vi "Handle Error.vi"(8 "error in (no error)":errorcluster, 11 "IMAQdx Actor in":refnum<class "IMAQdx Actor.lvclass">) -> (0 "error out":errorcluster, 2 "stop actor?":bool=TRUE, 3 "IMAQdx Actor out":refnum<class "IMAQdx Actor.lvclass">)   [LabVIEW 2020, in "IMAQdx Actor.lvlib" / "IMAQdx Actor.lvclass"]
doc: "(<B>Filename</B>: Actor Framework.lvlib:Actor.lvclass:Handle Error.vi)\n\nDefines how the actor handles an error that occurred while processing a message. By default, this method does nothing except stop the actor."
uses:
  IMAQdx Actor.lvclass
  C:/Users/AlexK/work/LabVIEW Programme/POLARIS CAM Log Abw und E/Submodules/HIJ Vision/Camera Actors/Camera Actor/Camera Actor/Camera Actor.lvclass
  C:/Program Files (x86)/National Instruments/LabVIEW 2020/vi.lib/ActorFramework/Actor/Actor.lvclass
  Camera Actor/Camera Actor/Camera Actor.lvclass/Camera Actor.ctl
  Camera Actor/Camera Actor/Operation Mode.ctl
  Report Error Msg Ex/Report Error Msg Ex.lvclass
  C:/Program Files (x86)/National Instruments/LabVIEW 2020/vi.lib/ActorFramework/Message/Message.lvclass
  <vilib>/ActorFramework/Actor/Actor.lvclass/Actor.ctl
  <vilib>/ActorFramework/Message Enqueuer/Message Enqueuer.lvclass/Message Enqueuer.ctl
  IMAQdx Actor.lvclass/IMAQdx Actor.ctl
  Camera Actor/Camera Actor/Read Camera State.vi
  Camera Actor/Camera Actor/Read Delay bw restarts.vi
  <vilib>/ActorFramework/Message Enqueuer/Init from Existing Queue.vi
  <vilib>/ActorFramework/Message Enqueuer/Message Enqueuer.lvclass
  Camera Actor/Camera Actor/Camera Actor.lvclass
  <vilib>/ActorFramework/Actor/Actor.lvclass
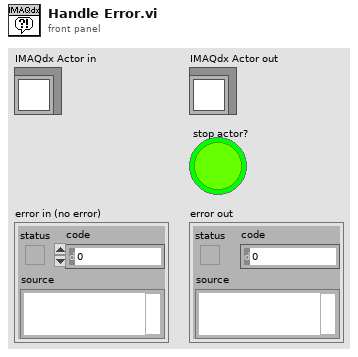
[diagram p1: front panel]
types:
  T1 = typedef "Camera Actor.lvlib/Camera Actor.lvclass/Operation Mode.ctl" = enum16{"Run", "Stop", "Exit", "Error", "Restart"}
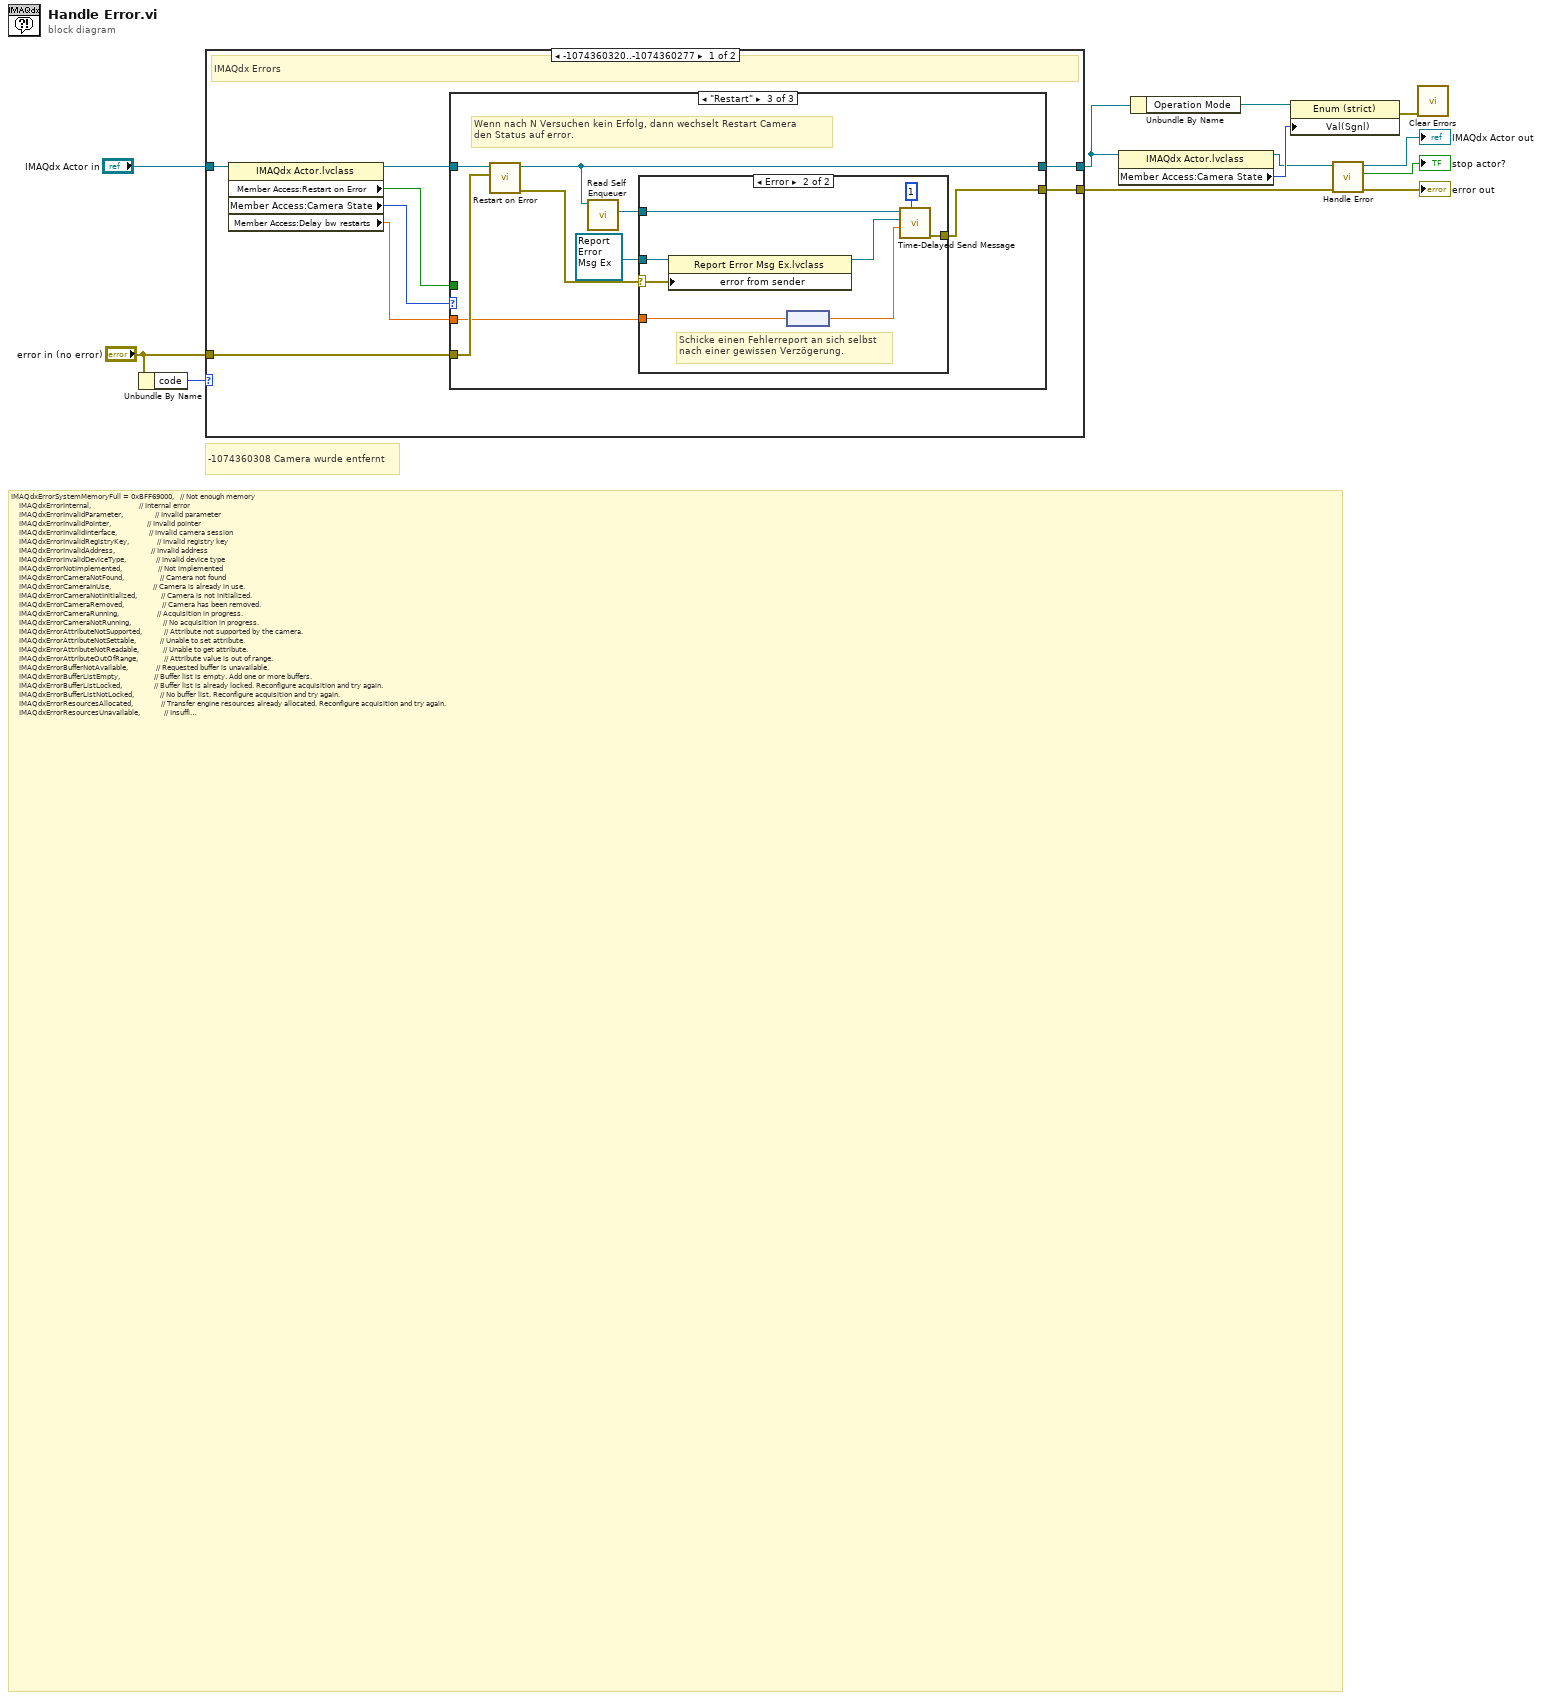
[diagram p0: block diagram]
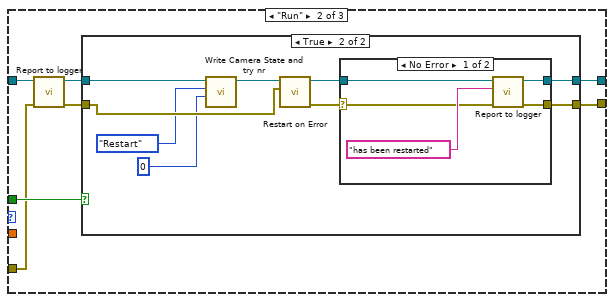
[diagram p3: hidden frame]
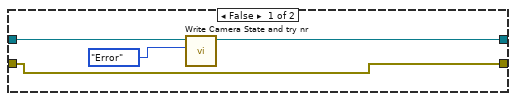
[diagram p4: hidden frame]
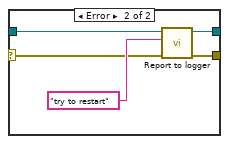
[diagram p5: hidden frame]
diagram:
  # "-1074360308 Camera wurde entfernt"
  # "IMAQdxErrorSystemMemoryFull = 0xBFF69000,   // Not enough memory\n    IMAQdxErrorInternal,                        // Internal error\n    IMAQdxErrorInvalidParameter,                // Invalid parameter\n    IMAQdxErrorInvalidPointer,                  // Invalid pointer\n    IMAQdxErrorInvalidInterface,                // Invalid camera session\n    IMAQdxErrorInvalidRegistryKey,              // Invalid registry key\n    IMAQdxErrorInvalidAddress,                  // Invalid address\n    IMAQdxErrorInvalidDeviceType,               // Invalid device type\n    IMAQdxErrorNotImplemented,                  // Not implemented\n    IMAQdxErrorCameraNotFound,                  // Camera not found\n    IMAQdxErrorCameraInUse,                     // Camera is already in use.\n    IMAQdxErrorCameraNotInitialized,            // Camera is not initialized.\n    IMAQdxErrorCameraRemoved,                   // Camera has been removed.\n    IMAQdxErrorCameraRunning,                   // Acquisition in progress.\n    IMAQdxErrorCameraNotRunning,                // No acquisition in progress.\n    IMAQdxErrorAttributeNotSupported,           // Attribute not supported by the camera.\n    IMAQdxErrorAttributeNotSettable,            // Unable to set attribute.\n    IMAQdxErrorAttributeNotReadable,            // Unable to get attribute.\n    IMAQdxErrorAttributeOutOfRange,             // Attribute value is out of range.\n    IMAQdxErrorBufferNotAvailable,              // Requested buffer is unavailable.\n    IMAQdxErrorBufferListEmpty,                 // Buffer list is empty. Add one or more buffers.\n    IMAQdxErrorBufferListLocked,                // Buffer list is already locked. Reconfigure acquisition and try again.\n    IMAQdxErrorBufferListNotLocked,             // No buffer list. Reconfigure acquisition and try again.\n    IMAQdxErrorResourcesAllocated,              // Transfer engine resources already allocated. Reconfigure acquisition and try again.\n    IMAQdxErrorResourcesUnavailable,            // Insufficient transfer engine resources.\n    IMAQdxErrorAsyncWrite,                      // Unable to perform asychronous register write.\n    IMAQdxErrorAsyncRead,                       // Unable to perform asychronous register read.\n    IMAQdxErrorTimeout,                         // Timeout.\n    IMAQdxErrorBusReset,                        // Bus reset occurred during a transaction.\n    IMAQdxErrorInvalidXML,                      // Unable to load camera's XML file.\n    IMAQdxErrorFileAccess,                      // Unable to read/write to file.\n    IMAQdxErrorInvalidCameraURLString,          // Camera has malformed URL string.\n    IMAQdxErrorInvalidCameraFile,               // Invalid camera file.\n    IMAQdxErrorGenICamError,                    // Unknown Genicam error.\n    IMAQdxErrorFormat7Parameters,               // For format 7: The combination of speed, image position, image size, and color coding is incorrect.\n    IMAQdxErrorInvalidAttributeType,            // The attribute type is not compatible with the passed variable type.\n    IMAQdxErrorDLLNotFound,                     // The DLL could not be found.\n    IMAQdxErrorFunctionNotFound,                // The function could not be found.\n    IMAQdxErrorLicenseNotActivated,             // License not activated.\n    IMAQdxErrorCameraNotConfiguredForListener,  // The camera is not configured properly to support a listener.\n    IMAQdxErrorCameraMulticastNotAvailable,     // Unable to configure the system for multicast support.\n    IMAQdxErrorBufferHasLostPackets,            // The requested buffer has lost packets and the user requested an error to be generated.\n    IMAQdxErrorGiGEVisionError,                 // Unknown GiGE Vision error.\n    IMAQdxErrorNetworkError,                    // Unknown network error.\n    IMAQdxErrorCameraUnreachable,               // Unable to connect to the camera.\n    IMAQdxErrorHighPerformanceNotSupported,     // High performance acquisition is not supported on the specified network interface. Connect the camera to a network interface running the high performance driver.\n    IMAQdxErrorInterfaceNotRenamed,             // Unable to rename interface. Invalid or duplicate name specified.\n    IMAQdxErrorNoSupportedVideoModes,           // The camera does not have any video modes which are supported.\n    IMAQdxErrorSoftwareTriggerOverrun,          // Software trigger overrun.\n    IMAQdxErrorTestPacketNotReceived,           // The system did not receive a test packet from the camera. The packet size may be too large for the network configuration or a firewall may be enabled.\n    IMAQdxErrorCorruptedImageReceived,          // The camera returned a corrupted image.\n    IMAQdxErrorCameraConfigurationHasChanged,   // The camera did not return an image of the correct type it was configured for previously.\n    IMAQdxErrorCameraInvalidAuthentication,     // The camera is configured with password authentication and either the user name and password were not configured or they are incorrect.\n    IMAQdxErrorUnknownHTTPError,                // The camera returned an unknown HTTP error.\n    IMAQdxErrorKernelDriverUnavailable,         // Unable to attach to the kernel mode driver.\n    IMAQdxErrorPixelFormatDecoderUnavailable,   // No decoder available for selected pixel format.\n    IMAQdxErrorFirmwareUpdateNeeded,            // The acquisition hardware needs a firmware update before it can be used.\n    IMAQdxErrorFirmwareUpdateRebootNeeded,      // The firmware on the acquisition hardware has been updated and the system must be rebooted before use.\n    IMAQdxErrorLightingCurrentOutOfRange,       // The requested current level from the lighting controller is not possible.\n    IMAQdxErrorUSB3VisionError,                 // Unknown USB3 Vision error.\n    IMAQdxErrorInvalidU3VUSBDescriptor,         // The camera has a USB descriptor that is incompatible with the USB3 Vision specification.\n    IMAQdxErrorU3VInvalidControlInterface,      // The USB3 Vision control interface is not implemented or is invalid on this camera.\n    IMAQdxErrorU3VControlInterfaceError,        // There was an error from the control interface of the USB3 Vision camera.\n    IMAQdxErrorU3VInvalidEventInterface,        // The USB3 Vision event interface is not implemented or is invalid on this camera.\n    IMAQdxErrorU3VEventInterfaceError,          // There was an error from the event interface of the USB3 Vision camera.\n    IMAQdxErrorU3VInvalidStreamInterface,       // The USB3 Vision stream interface is not implemented or is invalid on this camera.\n    IMAQdxErrorU3VStreamInterfaceError,         // There was an error from the stream interface of the USB3 Vision camera.\n    IMAQdxErrorU3VUnsupportedConnectionSpeed,   // The USB connection speed is not supported by the camera.  Check whether the camera is plugged into a USB 2.0 port instead of a USB 3.0 port.  If so, verify that the camera supports this use case.       \n    IMAQdxErrorU3VInsufficientPower,            // The USB3 Vision camera requires more current than can be supplied by the USB port in use.\n    IMAQdxErrorU3VInvalidMaxCurrent,            // The U3V_MaximumCurrentUSB20_mA registry value is not valid for the connected USB3 Vision camera.\n    IMAQdxErrorBufferIncompleteData,            // The requested buffer has incomplete data and the user requested an error to be generated.\n    IMAQdxErrorCameraAcquisitionConfigFailed,   // The camera returned an error starting the acquisition.\n    IMAQdxErrorCameraClosePending,              // The camera still has outstanding references and will be closed when these operations complete.\n    IMAQdxErrorSoftwareFault,                   // An unexpected software error occurred.\n    IMAQdxErrorCameraPropertyInvalid,           // The value for an invalid camera property was requested.\n    IMAQdxErrorJumboFramesNotEnabled,           // Jumbo frames are not enabled on the host.  Maximum packet size is 1500 bytes.\n    IMAQdxErrorBayerPixelFormatNotSelected,     // This operation requires that the camera has a Bayer pixel format selected."
  n1 = Unbundle By Name("error in (no error)") -> ("code"=w6:i32)
  n2 = case shown="-1074360320..-1074360277" w6 {
    tunnel: [w17 w71] -> w5
    tunnel: [w20 w70] -> w2
    tunnel: "error in (no error)" -> [w18 w71]
    tunnel: "IMAQdx Actor in" -> [w19 w70]
    frame -1074360320..-1074360277 {
      # "IMAQdx Errors"
      n3 = property class="IMAQdx Actor.lvclass"(reference=w19) -> (reference out=w16:refnum<class "IMAQdx Actor.lvclass">, "Member Access:Restart on Error"=w15:bool, "Member Access:Camera State"=w14:T1, "Member Access:Delay bw restarts"=w13:dbl[unit])  [unwired: 1 in, 1 out]
      n4 = case shown="\"Restart\"" w14 {
        tunnel: [w22 w28 w57] -> w20
        tunnel: w16 -> [w22 w29 w60]
        tunnel: w18 -> [w21 w24 w59]
        tunnel: w15 -> [_ w27 _]
        tunnel: [w21 w26 w53] -> w17
        tunnel: w13 -> [_ _ w54]
        frame "Error", Default {
        }
        frame "Run" {
          n5 = call-dynamic "Report to logger.vi"("error in (no error)"=w24, "Camera Actor in"=w29) -> ("error out"=w23:errorcluster, "Camera Actor out"=w25:refnum<class "IMAQdx Actor.lvclass">)  [unwired: 8 in]
          n6 = case shown="True" w27 {
            tunnel: w25 -> [w32 w36]
            tunnel: [w33 w40] -> w28
            tunnel: w23 -> [w30 w42]
            tunnel: [w30 w39] -> w26
            frame False {
              n7 = call-dynamic "Write Camera State and try nr.vi"("Operation Mode"=Operation_Mode."Error" ("Camera State"), "Camera Actor in"=w32) -> ("Camera Actor out"=w33:refnum<class "IMAQdx Actor.lvclass">)  [unwired: 9 in]
            }
            frame True {
              n8 = call-dynamic "Write Camera State and try nr.vi"("current try"=u8 0, "Operation Mode"=Operation_Mode."Restart" ("Camera State"), "Camera Actor in"=w36) -> ("Camera Actor out"=w37:refnum<class "IMAQdx Actor.lvclass">)  [unwired: 8 in]
              n9 = call-dynamic "Restart on Error.vi"("Camera error"=w42, "Camera Actor in"=w37) -> ("error out"=w38:errorcluster, "Camera Actor out"=w41:refnum<class "IMAQdx Actor.lvclass">)  [unwired: 8 in]
              n10 = case shown="No Error" w38 {
                selector: w38 -> [w44 w49]
                tunnel: w41 -> [w46 w51]
                tunnel: [w45 w50] -> w40
                tunnel: [w43 w48] -> w39
                frame No Error {
                  n11 = call-dynamic "Report to logger.vi"("error in (no error)"=w44, "Comment"="has been restarted", "Camera Actor in"=w46) -> ("error out"=w43:errorcluster, "Camera Actor out"=w45:refnum<class "IMAQdx Actor.lvclass">)  [unwired: 7 in]
                }
                frame Error {
                  n12 = call-dynamic "Report to logger.vi"("error in (no error)"=w49, "Comment"="try to restart", "Camera Actor in"=w51) -> ("error out"=w48:errorcluster, "Camera Actor out"=w50:refnum<class "IMAQdx Actor.lvclass">)  [unwired: 7 in]
                }
              }
            }
          }
        }
        frame "Restart" {
          # "Wenn nach N Versuchen kein Erfolg, dann wechselt Restart Camera \nden Status auf error."
          n13 = call-dynamic "Restart on Error.vi"("Camera error"=w59, "Camera Actor in"=w60) -> ("error out"=w58:errorcluster, "Camera Actor out"=w57:refnum<class "IMAQdx Actor.lvclass">)  [unwired: 8 in]
          n14 = call <vilib>:"Read Self Enqueuer.vi"("Actor"=w57) -> ("Self Enqueuer"=w56:refnum<class "Message Enqueuer.lvclass">)  [unwired: 10 in]
          n15 = case shown="Error" w58 {
            selector: w58 -> [w61 w65]
            tunnel: w56 -> [_ w69]
            tunnel: refnum<class "Report Error Msg Ex.lvclass"> refnum ("Report Error Msg Ex.lvclass") -> [_ w67]
            tunnel: w54 -> [_ w64]
            tunnel: [w61 w63] -> w53
            frame No Error {
            }
            frame Error {
              # "Schicke einen Fehlerreport an sich selbst\nnach einer gewissen Verzögerung."
              n16 = property class="Report Error Msg Ex.lvclass"(reference=w67, "error from sender"=w65) -> (reference out=w66:refnum<class "Report Error Msg Ex.lvclass">)  [unwired: 1 in, 1 out]
              n17 = node(w64) -> (w62:dbl)
              n18 = call <vilib>:"Time-Delayed Send Message.vi"("# Copies (0 = infinite repeat)"=u32 1, "Milliseconds To Wait"=w62, "Message"=w66, "Message Enqueuer"=w69) -> ("error out"=w63:errorcluster)  [unwired: 6 in, 1 out]
            }
          }
        }
      }
    }
    frame 0, Default {
    }
  }
  n19 = property class="IMAQdx Actor.lvclass"(reference=w2) -> (reference out=w3:refnum<class "IMAQdx Actor.lvclass">, "Member Access:Camera State"=w12:T1)  [unwired: 1 in, 1 out]
  n20 = Unbundle By Name(w2) -> ("Operation Mode"=w4:refnum<vi>)
  n21 = property class="Enum (strict)"(reference=w4, "Val(Sgnl)"=w12) -> (error out=w1:errorcluster)  [unwired: 1 in, 1 out]
  n22 = call-parent "Handle Error.vi"("error in (no error)"=w5, "Camera Actor in"=w3) -> ("error out"=→"error out":errorcluster, "stop actor?"=→"stop actor?":bool, "Camera Actor out"=→"IMAQdx Actor out":refnum<class "IMAQdx Actor.lvclass">)  [unwired: 7 in]
  n23 = call <vilib>:"Clear Errors.vi"("error in (no error)"=w1) -> ()  [unwired: 5 in, 2 out]
